vi "leybold QMH german.vi"() -> ()   [LabVIEW 2023]
uses:
  usr/local/natinst/LabVIEW-2023-64/examples/Design Patterns/Queued Message Handler/support/QMH Fundamentals - Message Cluster.ctl
  <vilib>/Instr/_visa.llb/VISA Configure Serial Port (Instr).vi
  global variables.vi
  <vilib>/Utility/error.llb/Error Cluster From Error Code.vi
  SubVI library/Send Graphite Metrics/Send Graphite Metrics.vi
  <vilib>/ErrorRing/Error Ring.xnode
panel:
  out "unsigned byte array":u8[](array[numeric])
  in  "Stop":bool
  in  "recipes":bool
  in  "Tab Control":T1(tab)
  out "REF Leistung (W)":i16
  in  "Vorwartsleistung (W)":bool=TRUE
  in  "CL":bool
  in  "CT":bool
  in  "RF Quelle":bool
  out "PFG600":string
  out "Antwort":string
  in  "+100":bool
  out "DC Spannung (V)":i16
  in  "Argon (SCCM)":bool
  in  "Sauerstioff (SCCM)":bool
  in  "Gas":bool
  in  "+10":bool
  in  "+1":bool
  in  "-1":bool
  in  "-10":bool
  in  "-100":bool
  in  "GAS Boost":bool
  in  "Timer":bool
  in  "Matchbox-Modus":bool
  in  "TimerOn":bool
  out "PR4000":string
  in  "P1":bool
  in  "P2":bool
  in  "P3":bool
  out "Endzeit":timestamp format="%<%H:%M:%S>T"
  out "Time":timestamp format="%<%H:%M:%S\n%x>T"
  in  "RS232":bool
  out "Waveform Chart":waveform(dbl)(graph)
  in  "1h":bool
  in  "8h":bool
  in  "24h":bool
  in  "All":bool
  out "Druck (mbar)":dbl format="%#_6e"
  # "GENERATOR"
  # "MFC"
  # "TIMER"
  # "VOREINSTELLUNGEN"
  # "DEBUG"
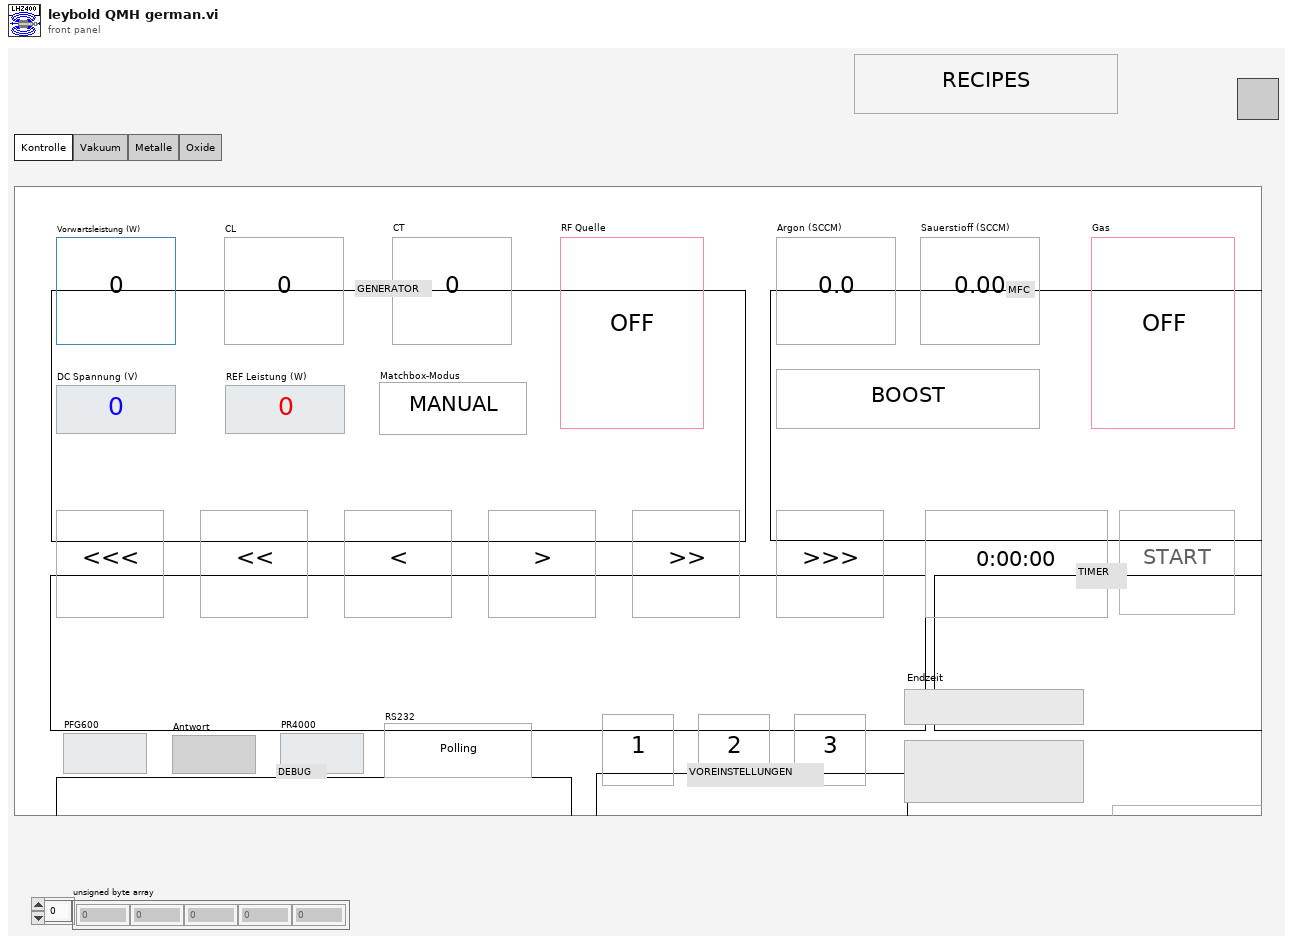
[diagram p1: front panel]
types:
  T1 = enum32{"Kontrolle", "Vakuum", "Metalle", "Oxide"}
  T2 = typedef "QMH Fundamentals - Message Cluster.ctl" = cluster{"Message":string, "Message Data":variant}
  T3 = cluster{"Message":string, enum16{"FWD", "CL", "CT", "Ar", "O2", "Timer"}}
  T4 = enum8{"Enabled", "Disabled", "Disabled and Grayed Out"}
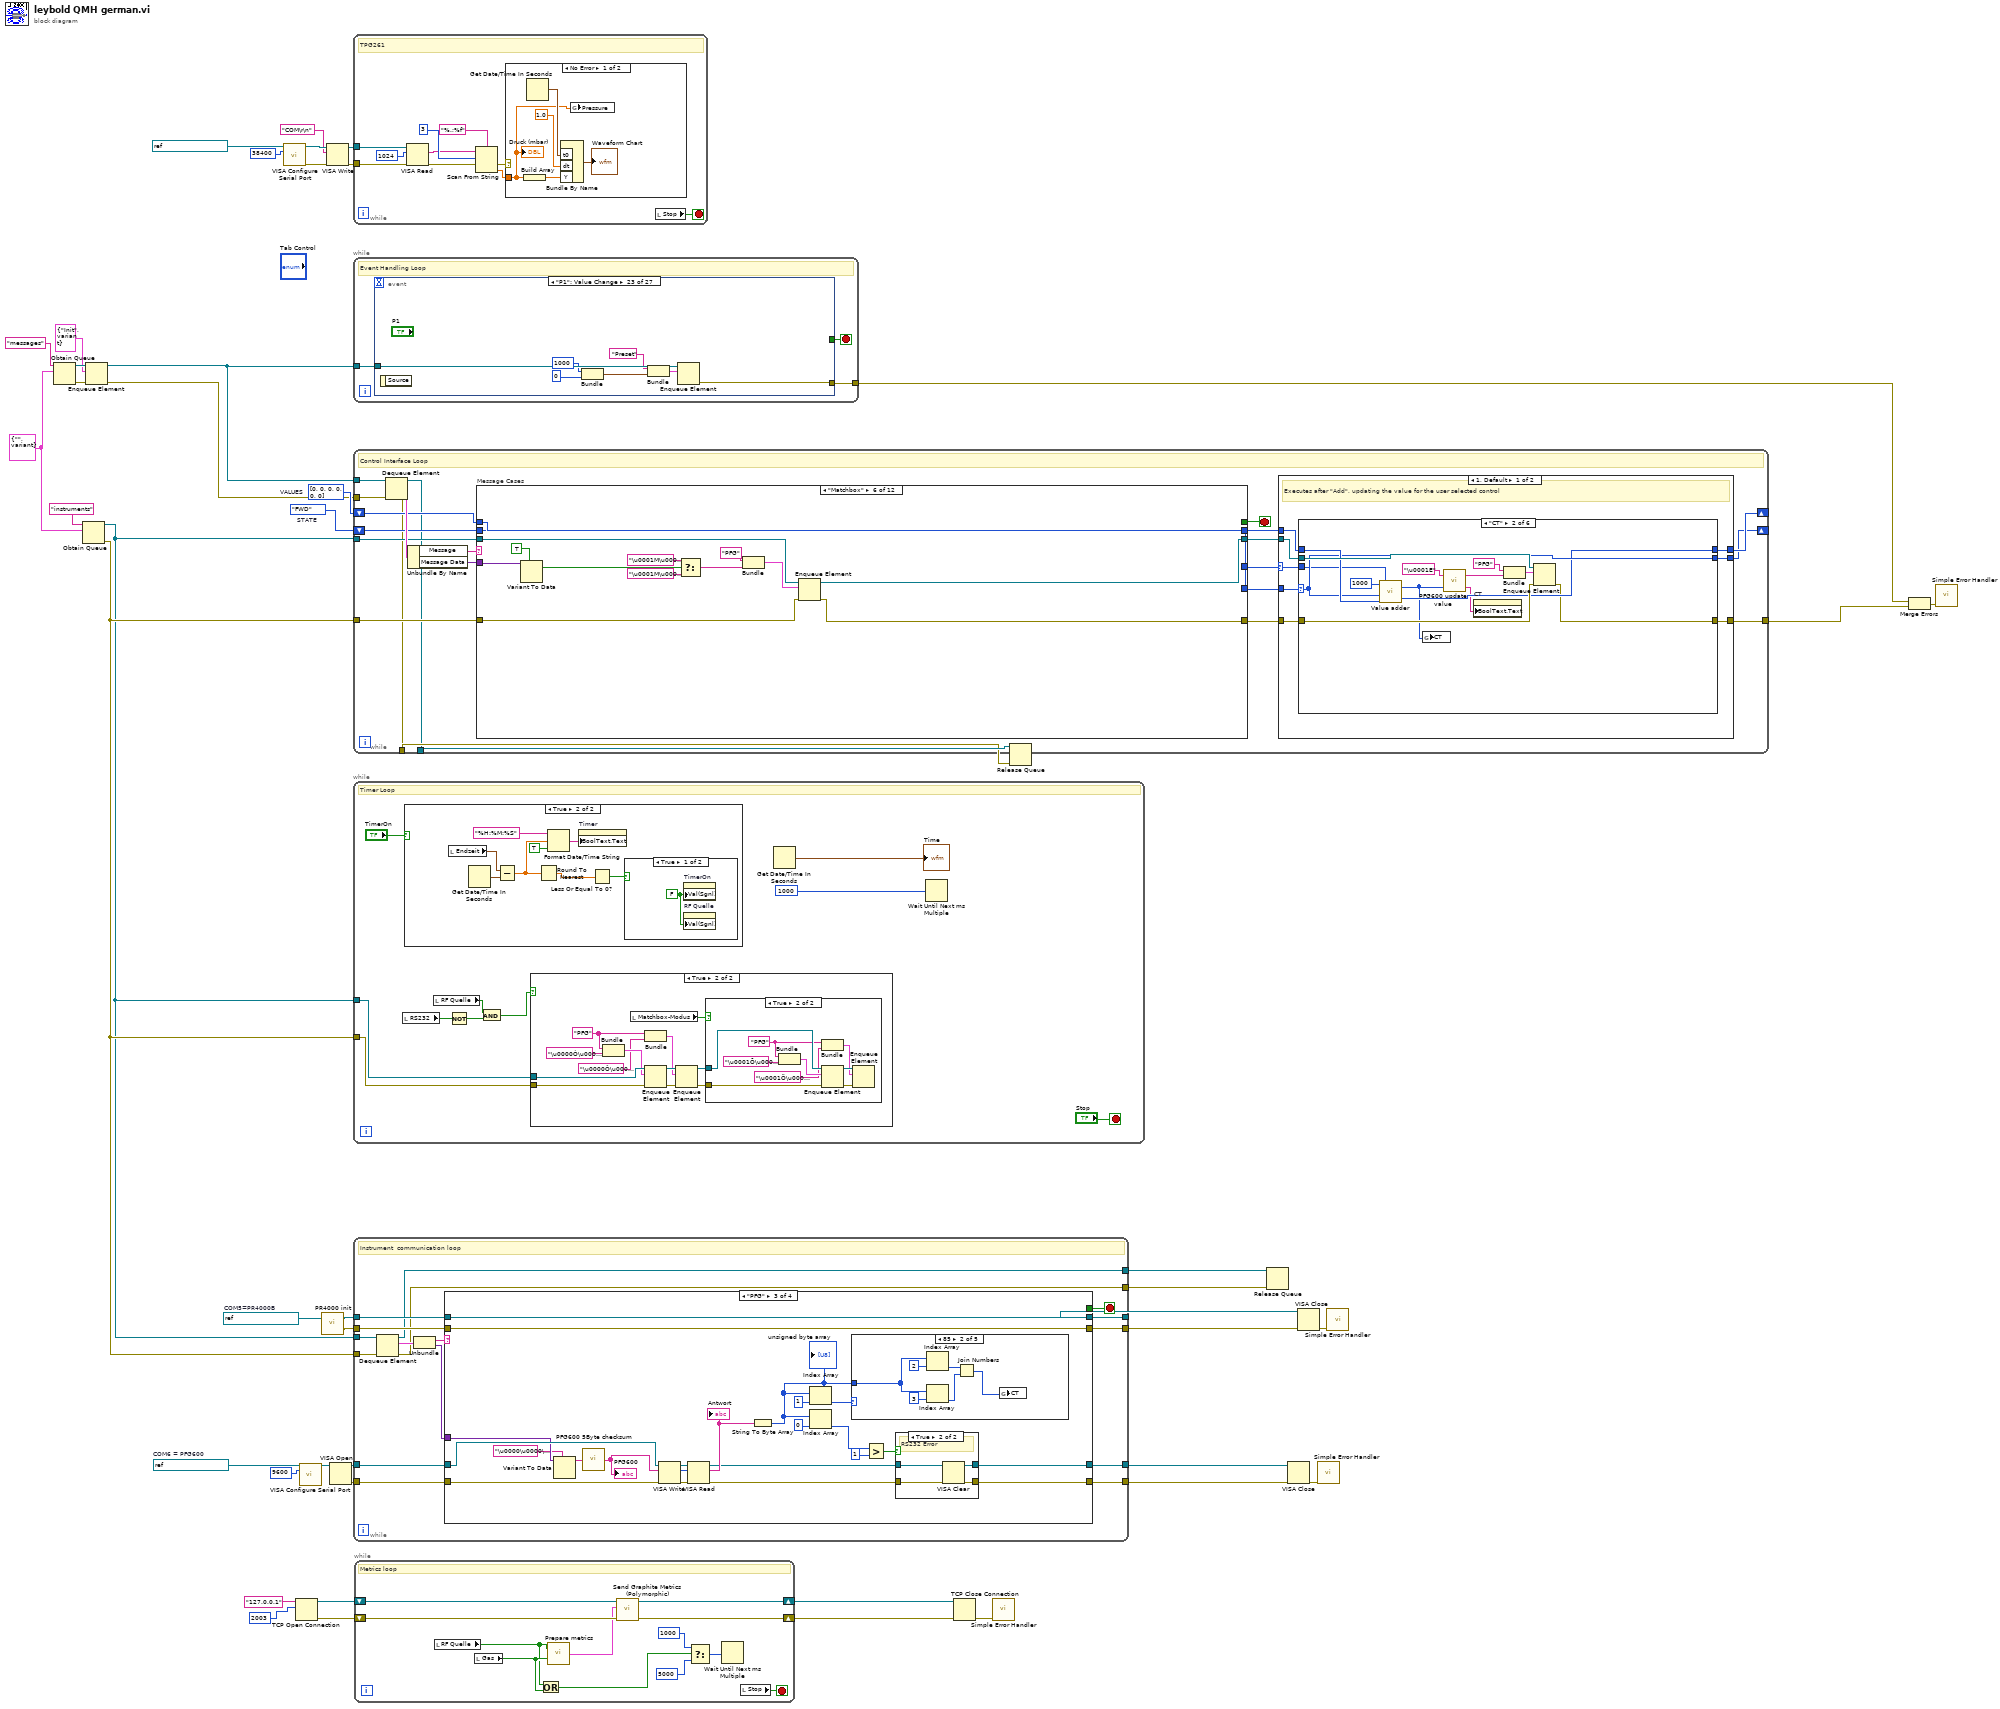
[diagram p0: block diagram]
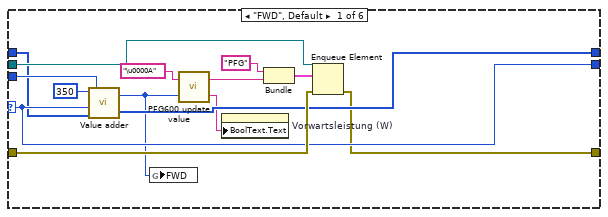
[diagram p6: hidden frame]
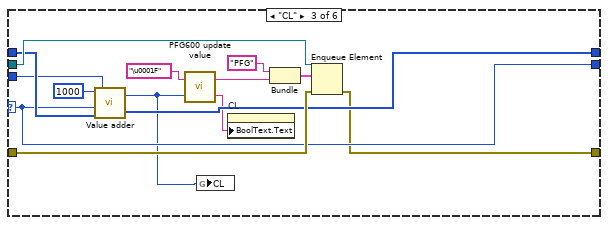
[diagram p7: hidden frame]
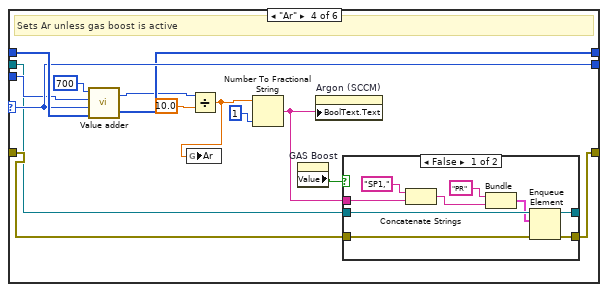
[diagram p8: hidden frame]
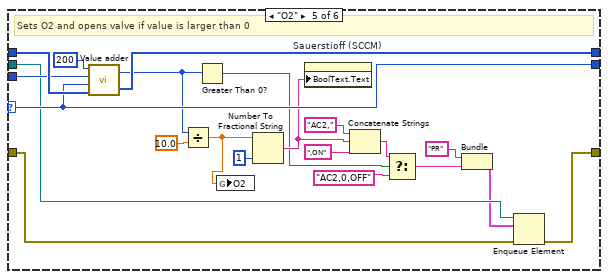
[diagram p10: hidden frame]
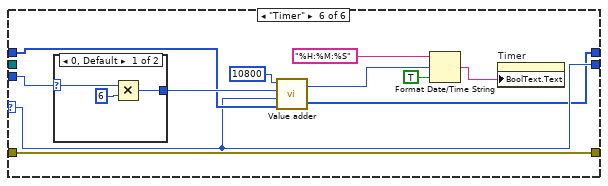
[diagram p11: hidden frame]
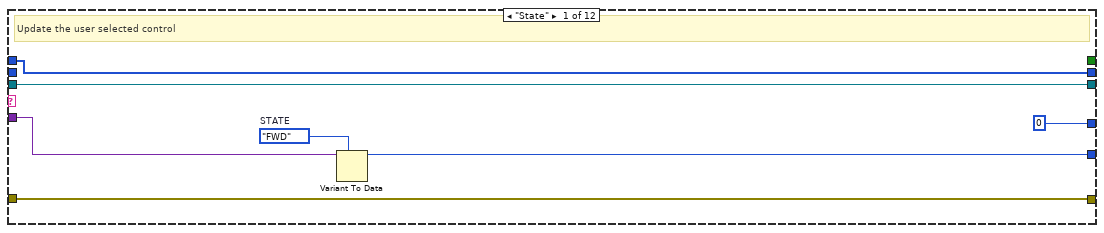
[diagram p14: hidden frame]
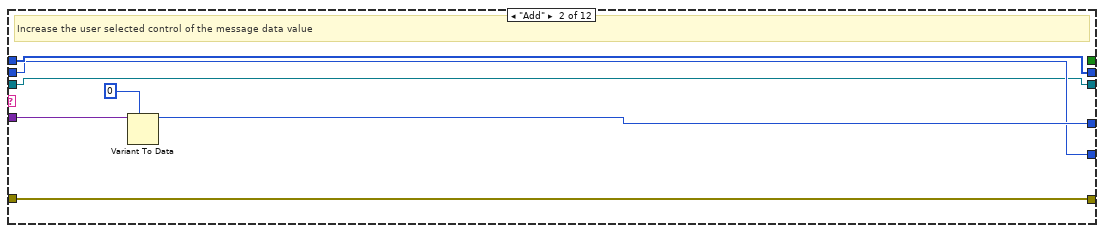
[diagram p15: hidden frame]
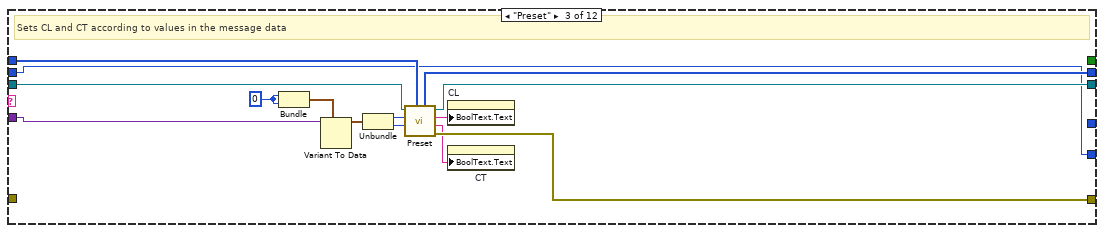
[diagram p16: hidden frame]
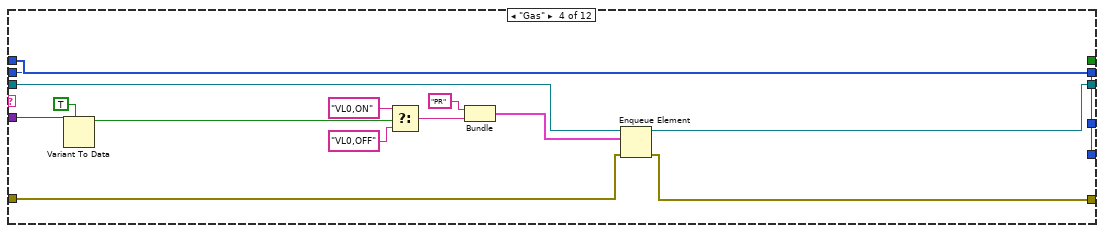
[diagram p17: hidden frame]
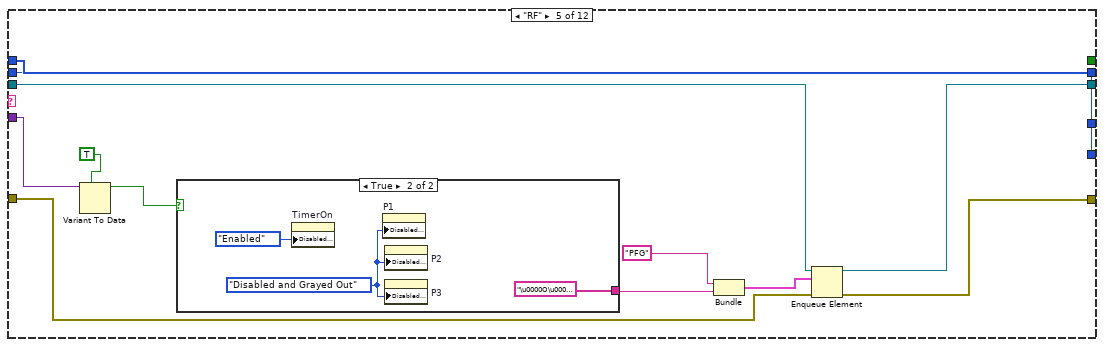
[diagram p18: hidden frame]
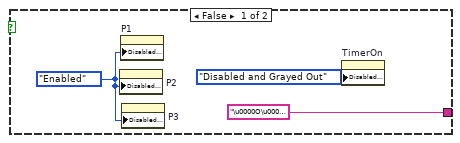
[diagram p19: hidden frame]
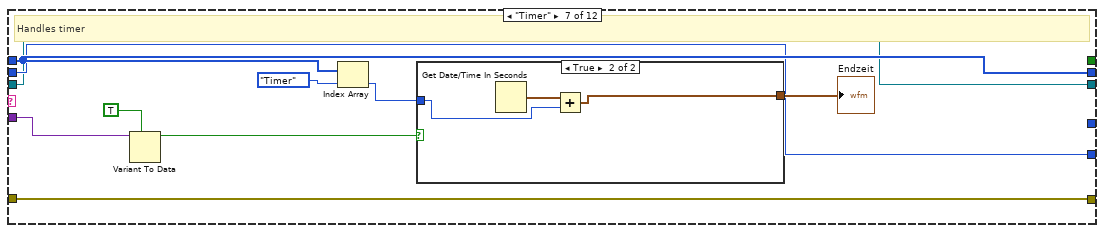
[diagram p20: hidden frame]
diagram:
  w27 = i16[] [0, 0, 0, 0, 0, 0]  # VALUES
  w28 = enum16{"FWD", "CL", "CT", "Ar", "O2", "Timer"}."FWD"  # STATE
  w19 = T2 {"Message"="", "Message Data"=variant} ("Message Cluster")
  w41 = refnum<visa-resource-name> "ASRL34::INSTR"  # COM5=PR4000B
  w15 = refnum<visa-resource-name> "ASRL36::INSTR"  # COM6 = PFG600
  n1 = Obtain Queue(name (unnamed)="messages", element data type=w19) -> (queue out=w32:refnum<queue>, error out=w33:errorcluster)  [unwired: 3 in, 1 out]
  n2 = Obtain Queue(name (unnamed)="instruments", element data type=w19) -> (queue out=w1:refnum<queue>, error out=w2:errorcluster)  [unwired: 3 in, 1 out]
  n3 = Enqueue Element(queue=w32, element=T2 {"Message"="Init", "Message Data"=variant}, error in (no error)=w33) -> (queue out=w26:refnum<queue>, error out=w10:errorcluster)  [unwired: 1 in, 1 out]
  n4 = call-poly "VISA Configure Serial Port"("VISA resource name"=refnum<visa-resource-name> "ASRL33::INSTR", "baud rate (9600)"=u32 38400) -> ("VISA resource name out"=w36:refnum<visa-resource-name>, "error out"=w37:errorcluster)  [unwired: 12 in]
  n5 = TCP Open Connection(address="127.0.0.1", remote port or service name=u16 2003) -> (connection ID=w7:refnum<k5>, error out=w6:errorcluster)  [unwired: 3 in]
  n6 = call-poly "VISA Configure Serial Port"("VISA resource name"=w15, "baud rate (9600)"=u32 9600) -> ("VISA resource name out"=w16:refnum<visa-resource-name>)  [unwired: 12 in, 1 out]
  n7 = call "PR4000 init.vi"("VISA Refnum in"=w41) -> ("error out"=w24:errorcluster, "VISA Refnum out"=w25:refnum<visa-resource-name>)  [unwired: 1 in]
  n8 = VISA Write(VISA resource name=w36, write buffer="COM\r\n", error in (no error)=w37) -> (VISA resource name out=w38:refnum<visa-resource-name>, error out=w34:errorcluster)  [unwired: 1 out]
  n9 = VISA Open(VISA resource name=w16) -> (VISA resource name=w46:refnum<visa-resource-name>, error out=w47:errorcluster)  [unwired: 4 in]
  n10 = while {
    tunnel: w38 -> [w57]
    tunnel: w34 -> [w56]
    stop <- w48 stop-if-true
    # "TPG261"
    n11 = VISA Read(VISA resource name=w57, byte count=u32 1024, error in (no error)=w56) -> (read buffer=w52:string, error out=w50:errorcluster)  [unwired: 2 out]
    n12 = Scan From String(format string="%.;%f" ("Format-String"), input string=w52, initial scan location=u32 3 ("offset (0)"), error in=w50) -> (error out=w49:errorcluster, output 1=w51:dbl)  [unwired: 1 in, 2 out]
    n13 = case shown="No Error" w49 {
      tunnel: w51 -> [w58 _]
      frame No Error {
        n14 = Build Array(w58) -> (w62:dbl[])
        n15 = Get Date/Time In Seconds() -> (seconds since 1Jan1904=w59:timestamp)
        n16 = Bundle By Name("t0"=w59, "dt"=1.0, "Y"=w62) -> (→"Waveform Chart":waveform(dbl))  [unwired: 1 in]
        n17 = global write "global variables.vi" "Pressure"(w58) -> ()
        "Druck (mbar)" <- w58
      }
      frame Error {
      }
    }
    n18 = local read "Stop"() -> (w48:bool)
  }
  n19 = while {
    tunnel: w26 -> [w65]
    tunnel: [w63] -> w30
    stop <- w64 stop-if-true
    # "Event Handling Loop"
    n20 = event shown="[22] \"P1\": Value Change" {
      selector: _ -> [_ _ _ _ _ _ _ _ _ _ _ _ _ _ _ _ _ _ _ _ _ _ _ _ _ _ _]
      dyn-events: _ -> [_ _ _ _ _ _ _ _ _ _ _ _ _ _ _ _ _ _ _ _ _ _ _ _ _ _ _]
      timeout: _ -> [_ _ _ _ _ _ _ _ _ _ _ _ _ _ _ _ _ _ _ _ _ _ _ _ _ _ _]
      tunnel: [TRUE _ _ _ _ _ _ _ _ _ _ _ _ _ _ _ _ _ _ _ _ _ _ _ _ _ _] -> w64
      tunnel: w65 -> [w69 w71 w76 w81 w86 w91 w98 w103 w108 w113 w118 w122 w125 w128 w131 w134 w137 w142 w147 _ w156 w160 w168 w175 w182 w187 _]
      tunnel: [w68 w70 w75 w80 w85 w90 w95 w100 w105 w110 w115 w121 w124 w127 w130 w133 w136 w141 w146 _ w152 w157 w162 w169 w176 w186 _] -> w63
      event "Stop": Value Change {
        # "Stop the VI."
        # "Enqueue an \"Exit\" message. Note that the Enqueue Element At Opposite End function is used to place this priority \"Exit\" message at the front of the queue ahead of all other messages."
        n21 = event-data() -> ()  [unwired: 1 in, 1 out]
        n22 = Enqueue Element At Opposite End(queue=w69, element=T2 {"Message"="Exit", "Message Data"=variant}) -> (error out=w68:errorcluster)  [unwired: 2 in, 2 out]
      }
      event "1h": Value Change {
        n23 = event-data() -> ()  [unwired: 1 in, 1 out]
        n24 = Bundle("Scale", 3600) -> (w73:cluster{string, i32})  [unwired: 1 in]
        n25 = Enqueue Element(queue=w71, element=w73) -> (error out=w70:errorcluster)  [unwired: 2 in, 2 out]
      }
      event "8h": Value Change {
        n26 = event-data() -> ()  [unwired: 1 in, 1 out]
        n27 = Bundle("Scale", 28800) -> (w78:cluster{string, i32})  [unwired: 1 in]
        n28 = Enqueue Element(queue=w76, element=w78) -> (error out=w75:errorcluster)  [unwired: 2 in, 2 out]
      }
      event "24h": Value Change {
        n29 = event-data() -> ()  [unwired: 1 in, 1 out]
        n30 = Bundle("Scale", 86400) -> (w83:cluster{string, i32})  [unwired: 1 in]
        n31 = Enqueue Element(queue=w81, element=w83) -> (error out=w80:errorcluster)  [unwired: 2 in, 2 out]
      }
      event "All": Value Change {
        n32 = event-data() -> ()  [unwired: 1 in, 1 out]
        n33 = Bundle("Scale", 0) -> (w88:cluster{string, i32})  [unwired: 1 in]
        n34 = Enqueue Element(queue=w86, element=w88) -> (error out=w85:errorcluster)  [unwired: 2 in, 2 out]
      }
      event "CL": Value Change {
        w94 = FALSE ("FWD Power (W)")
        n35 = event-data() -> ()  [unwired: 1 in, 1 out]
        n36 = Enqueue Element(queue=w91, element=T3 {"Message"="State", enum."CL"}) -> (error out=w90:errorcluster)  [unwired: 2 in, 2 out]
        n37 = property on="CT" class="Bool (strict)"("Value"=w94) -> ()  [unwired: 2 in, 2 out]
        n38 = property on="Timer" class="Bool (strict)"("Value"=w94) -> ()  [unwired: 2 in, 2 out]
        n39 = property on="CL" class="Bool (strict)"("Value"=TRUE ("CL")) -> ()  [unwired: 2 in, 2 out]
        n40 = property on="Argon (SCCM)" class="Bool (strict)"("Value"=w94) -> ()  [unwired: 2 in, 2 out]
        n41 = property on="Sauerstioff (SCCM)" class="Bool (strict)"("Value"=w94) -> ()  [unwired: 2 in, 2 out]
        n42 = property on="Vorwartsleistung (W)" class="Bool (strict)"("Value"=w94) -> ()  [unwired: 2 in, 2 out]
      }
      event "CT": Value Change {
        w97 = FALSE ("FWD Power (W)")
        n43 = event-data() -> ()  [unwired: 1 in, 1 out]
        n44 = Enqueue Element(queue=w98, element=T3 {"Message"="State", enum."CT"}) -> (error out=w95:errorcluster)  [unwired: 2 in, 2 out]
        n45 = property on="CT" class="Bool (strict)"("Value"=TRUE ("CL")) -> ()  [unwired: 2 in, 2 out]
        n46 = property on="CL" class="Bool (strict)"("Value"=w97) -> ()  [unwired: 2 in, 2 out]
        n47 = property on="Timer" class="Bool (strict)"("Value"=w97) -> ()  [unwired: 2 in, 2 out]
        n48 = property on="Argon (SCCM)" class="Bool (strict)"("Value"=w97) -> ()  [unwired: 2 in, 2 out]
        n49 = property on="Sauerstioff (SCCM)" class="Bool (strict)"("Value"=w97) -> ()  [unwired: 2 in, 2 out]
        n50 = property on="Vorwartsleistung (W)" class="Bool (strict)"("Value"=w97) -> ()  [unwired: 2 in, 2 out]
      }
      event "Argon (SCCM)": Value Change {
        w102 = FALSE ("FWD Power (W)")
        n51 = event-data() -> ()  [unwired: 1 in, 1 out]
        n52 = Enqueue Element(queue=w103, element=T3 {"Message"="State", enum."Ar"}) -> (error out=w100:errorcluster)  [unwired: 2 in, 2 out]
        n53 = property on="CL" class="Bool (strict)"("Value"=w102) -> ()  [unwired: 2 in, 2 out]
        n54 = property on="Argon (SCCM)" class="Bool (strict)"("Value"=TRUE ("CL")) -> ()  [unwired: 2 in, 2 out]
        n55 = property on="Timer" class="Bool (strict)"("Value"=w102) -> ()  [unwired: 2 in, 2 out]
        n56 = property on="CT" class="Bool (strict)"("Value"=w102) -> ()  [unwired: 2 in, 2 out]
        n57 = property on="Sauerstioff (SCCM)" class="Bool (strict)"("Value"=w102) -> ()  [unwired: 2 in, 2 out]
        n58 = property on="Vorwartsleistung (W)" class="Bool (strict)"("Value"=w102) -> ()  [unwired: 2 in, 2 out]
      }
      event "Sauerstioff (SCCM)": Value Change {
        w107 = FALSE ("FWD Power (W)")
        n59 = event-data() -> ()  [unwired: 1 in, 1 out]
        n60 = Enqueue Element(queue=w108, element=T3 {"Message"="State", enum."O2"}) -> (error out=w105:errorcluster)  [unwired: 2 in, 2 out]
        n61 = property on="CL" class="Bool (strict)"("Value"=w107) -> ()  [unwired: 2 in, 2 out]
        n62 = property on="Sauerstioff (SCCM)" class="Bool (strict)"("Value"=TRUE ("CL")) -> ()  [unwired: 2 in, 2 out]
        n63 = property on="Timer" class="Bool (strict)"("Value"=w107) -> ()  [unwired: 2 in, 2 out]
        n64 = property on="CT" class="Bool (strict)"("Value"=w107) -> ()  [unwired: 2 in, 2 out]
        n65 = property on="Argon (SCCM)" class="Bool (strict)"("Value"=w107) -> ()  [unwired: 2 in, 2 out]
        n66 = property on="Vorwartsleistung (W)" class="Bool (strict)"("Value"=w107) -> ()  [unwired: 2 in, 2 out]
      }
      event "Vorwartsleistung (W)": Value Change {
        w112 = FALSE ("FWD Power (W)")
        n67 = event-data() -> ()  [unwired: 1 in, 1 out]
        n68 = Enqueue Element(queue=w113, element=T3 {"Message"="State", enum."FWD"}) -> (error out=w110:errorcluster)  [unwired: 2 in, 2 out]
        n69 = property on="Vorwartsleistung (W)" class="Bool (strict)"("Value"=TRUE ("CL")) -> ()  [unwired: 2 in, 2 out]
        n70 = property on="Sauerstioff (SCCM)" class="Bool (strict)"("Value"=w112) -> ()  [unwired: 2 in, 2 out]
        n71 = property on="Timer" class="Bool (strict)"("Value"=w112) -> ()  [unwired: 2 in, 2 out]
        n72 = property on="CL" class="Bool (strict)"("Value"=w112) -> ()  [unwired: 2 in, 2 out]
        n73 = property on="Argon (SCCM)" class="Bool (strict)"("Value"=w112) -> ()  [unwired: 2 in, 2 out]
        n74 = property on="CT" class="Bool (strict)"("Value"=w112) -> ()  [unwired: 2 in, 2 out]
      }
      event "Timer": Value Change {
        w116 = FALSE ("FWD Power (W)")
        n75 = event-data() -> ()  [unwired: 1 in, 1 out]
        n76 = Enqueue Element(queue=w118, element=T3 {"Message"="State", enum."Timer"}) -> (error out=w115:errorcluster)  [unwired: 2 in, 2 out]
        n77 = property on="CT" class="Bool (strict)"("Value"=w116) -> ()  [unwired: 2 in, 2 out]
        n78 = property on="Timer" class="Bool (strict)"("Value"=TRUE ("CL")) -> ()  [unwired: 2 in, 2 out]
        n79 = property on="CL" class="Bool (strict)"("Value"=w116) -> ()  [unwired: 2 in, 2 out]
        n80 = property on="Argon (SCCM)" class="Bool (strict)"("Value"=w116) -> ()  [unwired: 2 in, 2 out]
        n81 = property on="Sauerstioff (SCCM)" class="Bool (strict)"("Value"=w116) -> ()  [unwired: 2 in, 2 out]
        n82 = property on="Vorwartsleistung (W)" class="Bool (strict)"("Value"=w116) -> ()  [unwired: 2 in, 2 out]
      }
      event "-100": Value Change {
        n83 = event-data() -> ()  [unwired: 1 in, 1 out]
        n84 = Enqueue Element(queue=w122, element=cluster{"Message":string, i32} {"Message"="Add", -100}) -> (error out=w121:errorcluster)  [unwired: 2 in, 2 out]
      }
      event "-10": Value Change {
        n85 = event-data() -> ()  [unwired: 1 in, 1 out]
        n86 = Enqueue Element(queue=w125, element=cluster{"Message":string, i32} {"Message"="Add", -10}) -> (error out=w124:errorcluster)  [unwired: 2 in, 2 out]
      }
      event "-1": Value Change {
        n87 = event-data() -> ()  [unwired: 1 in, 1 out]
        n88 = Enqueue Element(queue=w128, element=cluster{"Message":string, i32} {"Message"="Add", -1}) -> (error out=w127:errorcluster)  [unwired: 2 in, 2 out]
      }
      event "+1": Value Change {
        n89 = event-data() -> ()  [unwired: 1 in, 1 out]
        n90 = Enqueue Element(queue=w131, element=cluster{"Message":string, i32} {"Message"="Add", 1}) -> (error out=w130:errorcluster)  [unwired: 2 in, 2 out]
      }
      event "+10": Value Change {
        n91 = event-data() -> ()  [unwired: 1 in, 1 out]
        n92 = Enqueue Element(queue=w134, element=cluster{"Message":string, i32} {"Message"="Add", 10}) -> (error out=w133:errorcluster)  [unwired: 2 in, 2 out]
      }
      event "+100": Value Change {
        n93 = event-data() -> ()  [unwired: 1 in, 1 out]
        n94 = Enqueue Element(queue=w137, element=cluster{"Message":string, i32} {"Message"="Add", 100}) -> (error out=w136:errorcluster)  [unwired: 2 in, 2 out]
      }
      event "GAS Boost": Value Change {
        n95 = event-data() -> ()  [unwired: 1 in, 1 out]
        n96 = Bundle("Message"="Boost", "GAS Boost"="GAS Boost") -> (w138:cluster{"Message":string, "GAS Boost":bool})  [unwired: 1 in]
        n97 = Enqueue Element(queue=w142, element=w138) -> (error out=w141:errorcluster)  [unwired: 2 in, 2 out]
      }
      event "Gas": Value Change {
        n98 = event-data() -> ()  [unwired: 1 in, 1 out]
        n99 = Bundle("Gas", "Gas"="Gas") -> (w145:cluster{string, "Gas":bool})  [unwired: 1 in]
        n100 = Enqueue Element(queue=w147, element=w145) -> (error out=w146:errorcluster)  [unwired: 2 in, 2 out]
      }
      event "RS232": Value Change {
        n101 = event-data() -> ()  [unwired: 1 in, 1 out]
        n102 = case shown="True" "RS232" {
          tunnel: [T4."Enabled" ("Disabled") T4."Disabled and Grayed Out" ("Disabled")] -> w148
          frame False {
          }
          frame True {
          }
        }
        n103 = property on="DC Spannung (V)" class="DigNum (strict)"("DisabledEnum"=w148) -> ()  [unwired: 2 in, 2 out]
        n104 = property on="REF Leistung (W)" class="DigNum (strict)"("DisabledEnum"=w148) -> ()  [unwired: 2 in, 2 out]
      }
      event "TimerOn": Value Change {
        n105 = event-data() -> ("NewVal"=w155:bool)  [unwired: 1 in]
        n106 = Bundle("Timer", "NewVal"=w155) -> (w153:cluster{string, "NewVal":bool})  [unwired: 1 in]
        n107 = Enqueue Element(queue=w156, element=w153) -> (error out=w152:errorcluster)  [unwired: 2 in, 2 out]
      }
      event "RF Quelle": Value Change {
        n108 = event-data() -> ()  [unwired: 1 in, 1 out]
        n109 = Bundle("RF", "RF Quelle"="RF Quelle") -> (w159:cluster{string, "RF Quelle":bool})  [unwired: 1 in]
        n110 = Enqueue Element(queue=w160, element=w159) -> (error out=w157:errorcluster)  [unwired: 2 in, 2 out]
      }
      event "P1": Value Change {
        n111 = event-data() -> ()  [unwired: 1 in, 1 out]
        n112 = Bundle(1000, 0) -> (w165:cluster{i32, i32})  [unwired: 1 in]
        n113 = Bundle("Preset", w165) -> (w166:cluster{string, cluster{i32, i32}})  [unwired: 1 in]
        n114 = Enqueue Element(queue=w168, element=w166) -> (error out=w162:errorcluster)  [unwired: 2 in, 2 out]
      }
      event "P2": Value Change {
        n115 = event-data() -> ()  [unwired: 1 in, 1 out]
        n116 = Bundle(250, 750) -> (w172:cluster{i32, i32})  [unwired: 1 in]
        n117 = Bundle("Preset", w172) -> (w173:cluster{string, cluster{i32, i32}})  [unwired: 1 in]
        n118 = Enqueue Element(queue=w175, element=w173) -> (error out=w169:errorcluster)  [unwired: 2 in, 2 out]
      }
      event "P3": Value Change {
        n119 = event-data() -> ()  [unwired: 1 in, 1 out]
        n120 = Bundle(680, 580) -> (w179:cluster{i32, i32})  [unwired: 1 in]
        n121 = Bundle("Preset", w179) -> (w180:cluster{string, cluster{i32, i32}})  [unwired: 1 in]
        n122 = Enqueue Element(queue=w182, element=w180) -> (error out=w176:errorcluster)  [unwired: 2 in, 2 out]
      }
      event "Matchbox-Modus": Value Change {
        n123 = event-data() -> ()  [unwired: 1 in, 1 out]
        n124 = Bundle("Matchbox", "Matchbox-Modus"="Matchbox-Modus") -> (w183:cluster{string, "Matchbox-Modus":bool})  [unwired: 1 in]
        n125 = Enqueue Element(queue=w187, element=w183) -> (error out=w186:errorcluster)  [unwired: 2 in, 2 out]
      }
      event "recipes": Value Change {
        n126 = event-data() -> ()  [unwired: 1 in, 1 out]
        n127 = call <vilib>:"System Exec.vi"("wait until completion? (T)"=FALSE, "command line"="firefox https://docs.google.com/spreadsheets/d/1f53240c20IwFszMSA94HhWp93EeL4Y7tCwhda4_pTaQ/edit#gid=1759381600 ") -> ()  [unwired: 6 in, 4 out]
      }
    }
  }
  n128 = while {
    tunnel: w26 -> [w206]
    tunnel: w10 -> [w205]
    shift-right: [w202] -> _
    shift-left: w27 -> [w201]
    shift-right: [w196] -> _
    shift-left: w28 -> [w204]
    tunnel: w1 -> [w195]
    tunnel: [w193] -> w18
    tunnel: w2 -> [w192]
    tunnel: [w191] -> w14
    tunnel: [w190] -> w13
    stop <- w194 stop-if-true
    # "Control Interface Loop"
    n129 = Dequeue Element(queue=w206, error in (no error)=w205) -> (queue out=w191:refnum<queue>, element=w209:T2, error out=w190:errorcluster)  [unwired: 1 in, 1 out]
    n130 = Unbundle By Name(w209) -> ("Message"=w208:string, "Message Data"=w207:variant)
    n131 = case "Message Cases" shown="\"Matchbox\"" w208 {
      selector: w208 -> [_ _ _ _ _ _ _ _ _ w450 _ w472]
      tunnel: w207 -> [w330 w337 w351 w361 w369 w389 w403 w426 _ w449 w464 _]
      tunnel: [w327 w334 w342 w365 w377 w397 w401 w424 w446 w456 w470 w476] -> w198
      tunnel: w204 -> [_ w333 w339 w364 w376 w396 w400 w417 w445 w455 w467 w475]
      tunnel: [0 w335 _ _ _ _ _ 0 _ _ _ 0] -> w203
      tunnel: w201 -> [w327 w334 w343 w365 w377 w397 w401 w424 w446 w456 w470 w476]
      tunnel: [w325 w332 w345 w357 w370 w393 w399 w420 w444 w453 w469 w474] -> w200
      tunnel: [w324 w331 w344 w362 w371 w392 w398 w419 w438 w447 w468 w471] -> w199
      tunnel: [w326 w333 w339 w364 w376 w396 w400 w417 w445 w455 w467 w475] -> w197
      tunnel: w195 -> [w325 w332 w338 w363 w372 w394 w399 w416 w444 w452 w469 w474]
      tunnel: [_ _ _ _ _ _ _ _ _ TRUE _ _] -> w194
      tunnel: w192 -> [w324 w331 _ w356 w366 w388 w398 _ w438 w448 w468 w471]
      frame "State" {
        w328 = enum16{"FWD", "CL", "CT", "Ar", "O2", "Timer"}."FWD"  # STATE
        # "Update the user selected control"
        n132 = Variant To Data(type=w328, Variant=w330) -> (data=w326:enum16{"FWD", "CL", "CT", "Ar", "O2", "Timer"})  [unwired: 1 in, 1 out]
      }
      frame "Add" {
        # "Increase the user selected control of the message data value"
        n133 = Variant To Data(type=0, Variant=w337) -> (data=w335:i32)  [unwired: 1 in, 1 out]
      }
      frame "Preset" {
        w350 = 0
        # "Sets CL and CT according to values in the message data"
        n134 = Bundle(w350, w350) -> (w349:cluster{i32, i32})  [unwired: 1 in]
        n135 = Variant To Data(type=w349, Variant=w351) -> (data=w348:cluster{i32, i32})  [unwired: 1 in, 1 out]
        n136 = Unbundle(w348) -> (w347:i32, w346:i32)
        n137 = call "Preset.vi"("Array"=w343, "CT"=w346, "CL"=w347, "queue in"=w338) -> ("error out"=w344:errorcluster, "Text CT"=w340:string, "Text CL"=w341:string, "queue out"=w345:refnum<queue>, "output array"=w342:i16[])  [unwired: 3 in]
        n138 = property on="CL" class="Bool (strict)"("BoolText.Text"=w341) -> ()  [unwired: 2 in, 2 out]
        n139 = property on="CT" class="Bool (strict)"("BoolText.Text"=w340) -> ()  [unwired: 2 in, 2 out]
      }
      frame "Gas" {
        n140 = Variant To Data(type=TRUE, Variant=w361) -> (data=w355:bool)  [unwired: 1 in, 1 out]
        n141 = Select(t="VL0,ON" ("string"), s=w355, f="VL0,OFF" ("string")) -> (s? t:f=w352:string)
        n142 = Bundle("PR", "string"=w352) -> (w358:cluster{string, "string":string})  [unwired: 1 in]
        n143 = Enqueue Element(queue=w363, element=w358, error in (no error)=w356) -> (queue out=w357:refnum<queue>, error out=w362:errorcluster)  [unwired: 1 in, 1 out]
      }
      frame "RF" {
        n144 = Variant To Data(type=TRUE, Variant=w369) -> (data=w367:bool)  [unwired: 1 in, 1 out]
        n145 = case shown="True" w367 {
          tunnel: ["\u0000O\u0000\u0000" "\u0000O\u0000\u0001"] -> w375
          frame False {
            w378 = T4."Enabled" ("Disabled")
            n146 = property on="P2" class="Bool"("DisabledEnum"=w378) -> ()  [unwired: 2 in, 2 out]
            n147 = property on="P1" class="Bool"("DisabledEnum"=w378) -> ()  [unwired: 2 in, 2 out]
            n148 = property on="P3" class="Bool"("DisabledEnum"=w378) -> ()  [unwired: 2 in, 2 out]
            n149 = property on="TimerOn" class="Bool (strict)"("DisabledEnum"=T4."Disabled and Grayed Out" ("Disabled")) -> ()  [unwired: 2 in, 2 out]
          }
          frame True {
            w381 = T4."Disabled and Grayed Out" ("Disabled")
            n150 = property on="TimerOn" class="Bool (strict)"("DisabledEnum"=T4."Enabled" ("Disabled")) -> ()  [unwired: 2 in, 2 out]
            n151 = property on="P1" class="Bool"("DisabledEnum"=w381) -> ()  [unwired: 2 in, 2 out]
            n152 = property on="P2" class="Bool"("DisabledEnum"=w381) -> ()  [unwired: 2 in, 2 out]
            n153 = property on="P3" class="Bool"("DisabledEnum"=w381) -> ()  [unwired: 2 in, 2 out]
          }
        }
        n154 = Bundle("PFG", w375) -> (w373:cluster{string, string})  [unwired: 1 in]
        n155 = Enqueue Element(queue=w372, element=w373, error in (no error)=w366) -> (queue out=w370:refnum<queue>, error out=w371:errorcluster)  [unwired: 1 in, 1 out]
      }
      frame "Matchbox" {
        n156 = Variant To Data(type=TRUE, Variant=w389) -> (data=w387:bool)  [unwired: 1 in, 1 out]
        n157 = Select(t="\u0001M\u0000\u0002", s=w387, f="\u0001M\u0000\u0001") -> (s? t:f=w384:string)
        n158 = Bundle("PFG", w384) -> (w391:cluster{string, string})  [unwired: 1 in]
        n159 = Enqueue Element(queue=w394, element=w391, error in (no error)=w388) -> (queue out=w393:refnum<queue>, error out=w392:errorcluster)  [unwired: 1 in, 1 out]
      }
      frame "Timer" {
        # "Handles timer"
        n160 = Variant To Data(type=TRUE, Variant=w403) -> (data=w402:bool)  [unwired: 1 in, 1 out]
        n161 = Index Array(array=w401, index=enum16{"FWD", "CL", "CT", "Ar", "O2", "Timer"}."Timer") -> (element=w406:i16)
        n162 = case shown="True" w402 {
          tunnel: w406 -> [w408 w413]
          tunnel: [timestamp(0 s since 1904-01-01) w414] -> w407
          frame False {
            n163 = Format Date/Time String(time format string (%c)="%H:%M:%S", seconds (now)=w408, UTC format=TRUE) -> (date/time string=w409:string)
            n164 = property on="Timer" class="Bool (strict)"("BoolText.Text"=w409) -> ()  [unwired: 2 in, 2 out]
          }
          frame True {
            n165 = Get Date/Time In Seconds() -> (seconds since 1Jan1904=w415:timestamp)
            n166 = Add(x=w415, y=w413) -> (x+y=w414:timestamp)
          }
        }
        "Endzeit" <- w407
      }
      frame "Boost" {
        # "Sets Ar to 60 SCCM or revert to previous value"
        n167 = Variant To Data(type=TRUE, Variant=w426) -> (data=w418:bool)  [unwired: 1 in, 1 out]
        n168 = case shown="False" w418 {
          tunnel: [w433 "SP1,60.0"] -> w422
          tunnel: w424 -> [w436 _]
          frame False {
            n169 = Index Array(array=w436, index=enum16{"FWD", "CL", "CT", "Ar", "O2", "Timer"}."Ar") -> (element=w430:i16)
            n170 = Divide(x=w430, y=10.0) -> (x/y=w429:dbl)
            n171 = Number To Fractional String(number=w429, precision (6)=i16 1) -> (F-format string=w431:string)  [unwired: 2 in]
            n172 = Concatenate Strings("SP1," ("string"), w431) -> (w433:string)
          }
          frame True {
          }
        }
        n173 = Bundle("PR", w422) -> (w421:cluster{string, string})  [unwired: 1 in]
        n174 = Enqueue Element(queue=w416, element=w421) -> (queue out=w420:refnum<queue>, error out=w419:errorcluster)  [unwired: 2 in, 1 out]
      }
      frame "Init" {
        w439 = "0" ("Boolean Text.Text")
        # "Interface initzialization"
        n175 = property on="Tab Control" class="TabCtl (strict)"("TabHeight"=u32 50 ("Fixed Tab Dimension:Height")) -> ()  [unwired: 2 in, 2 out]
        n176 = property on="CL" class="Bool (strict)"("BoolText.Text"=w439) -> ()  [unwired: 2 in, 2 out]
        n177 = property on="Vorwartsleistung (W)" class="Bool (strict)"("BoolText.Text"=w439) -> ()  [unwired: 2 in, 2 out]
        n178 = property on="CT" class="Bool (strict)"("BoolText.Text"=w439) -> ()  [unwired: 2 in, 2 out]
        n179 = property on="Argon (SCCM)" class="Bool (strict)"("BoolText.Text"="0.0") -> ()  [unwired: 2 in, 2 out]
        n180 = invoke class="VI" method="Default Vals.Reinit All"() -> ()  [unwired: 3 in, 3 out]
        n181 = property on="Sauerstioff (SCCM)" class="Bool (strict)"("BoolText.Text"="0.00") -> ()  [unwired: 2 in, 2 out]
        n182 = property on="Timer" class="Bool (strict)"("BoolText.Text"="0:00:00" ("Boolean Text.Text")) -> ()  [unwired: 2 in, 2 out]
      }
      frame "Exit" {
        # "Stop the VI."
        # "Releases Queue and exit"
        n183 = Bundle(w450, "Message Data"=w449) -> (w451:cluster{string, "Message Data":variant})  [unwired: 1 in]
        n184 = Enqueue Element(queue=w452, element=w451, error in (no error)=w448) -> (queue out=w453:refnum<queue>, error out=w447:errorcluster)  [unwired: 1 in, 1 out]
      }
      frame "Scale" {
        n185 = Variant To Data(type=0, Variant=w464) -> (data=w460:i32)  [unwired: 1 in, 1 out]
        n186 = Get Date/Time In Seconds() -> (seconds since 1Jan1904=w466:timestamp)
        n187 = Equal To 0?(x=w460) -> (x = 0?=w461:bool)
        n188 = To Double Precision Float(number=w466) -> (double precision float=w465:dbl)
        n189 = Select(t=2, s=w461, f=0) -> (s? t:f=w459:i32)
        n190 = Subtract(x=w465, y=w460) -> (x-y=w462:dbl)
        n191 = property on="Waveform Chart" class="WFChart (strict)"("XScale.Maximum"=w465, "XScale.Minimum"=w462, "XScale.ScaleFit"=w459) -> ()  [unwired: 2 in, 2 out]
      }
      frame Default {
        # "Case not handled"
        n192 = xnode "Error Ring"("parameter 0"=w472) -> ("error out"=w473:errorcluster)
        n193 = call <vilib>:"Simple Error Handler.vi"("error in (no error)"=w473) -> ()  [unwired: 4 in, 5 out]
      }
    }
    n194 = case shown="1, Default" w203 {
      selector: w203 -> [w213 _]
      tunnel: w199 -> [w215 w321]
      tunnel: w198 -> [w217 w323]
      tunnel: [w216 w323] -> w202
      tunnel: w200 -> [w214 _]
      tunnel: w197 -> [w212 w322]
      tunnel: [w211 w322] -> w196
      tunnel: [w210 w321] -> w193
      frame 1, Default {
        # "Executes after \"Add\", updating the value for the user selected control"
        n195 = case shown="\"CT\"" w212 {
          selector: w212 -> [w226 w240 w254 w271 w303 w313]
          tunnel: [w226 w240 w254 w271 w303 w313] -> w211
          tunnel: w217 -> [w225 w241 w255 w272 w304 w314]
          tunnel: w213 -> [w227 w239 w253 w270 w302 w311]
          tunnel: [w224 w238 w252 w269 w301 w312] -> w216
          tunnel: w214 -> [w230 w244 w258 w262 w297 _]
          tunnel: w215 -> [w229 w243 w257 w265 w298 w306]
          tunnel: [w219 w233 w247 w261 w293 w306] -> w210
          frame "FWD", Default {
            n196 = call "Value adder.vi"("Array"=w225, "Enum"=w226, "value"=w227, "Max Limit"=i16 350) -> ("output array"=w224:i16[], "Limited value"=w218:i16)
            n197 = global write "global variables.vi" "FWD"(w218) -> ()
            n198 = call "PFG600 update value.vi"("Value"=w218, "Command"="\u0000A") -> ("Text"=w223:string, "Hex"=w222:string)
            n199 = property on="Vorwartsleistung (W)" class="Bool (strict)"("BoolText.Text"=w223) -> ()  [unwired: 2 in, 2 out]
            n200 = Bundle("PFG", "Hex"=w222) -> (w220:cluster{string, "Hex":string})  [unwired: 1 in]
            n201 = Enqueue Element(queue=w230, element=w220, error in (no error)=w229) -> (error out=w219:errorcluster)  [unwired: 1 in, 2 out]
          }
          frame "CT" {
            n202 = call "Value adder.vi"("Array"=w241, "Enum"=w240, "value"=w239, "Max Limit"=i16 1000) -> ("output array"=w238:i16[], "Limited value"=w232:i16)
            n203 = global write "global variables.vi" "CT"(w232) -> ()
            n204 = call "PFG600 update value.vi"("Value"=w232, "Command"="\u0001E") -> ("Text"=w237:string, "Hex"=w235:string)
            n205 = property on="CT" class="Bool (strict)"("BoolText.Text"=w237) -> ()  [unwired: 2 in, 2 out]
            n206 = Bundle("PFG", "Hex"=w235) -> (w234:cluster{string, "Hex":string})  [unwired: 1 in]
            n207 = Enqueue Element(queue=w244, element=w234, error in (no error)=w243) -> (error out=w233:errorcluster)  [unwired: 1 in, 2 out]
          }
          frame "CL" {
            n208 = call "Value adder.vi"("Array"=w255, "Enum"=w254, "value"=w253, "Max Limit"=i16 1000) -> ("output array"=w252:i16[], "Limited value"=w246:i16)
            n209 = call "PFG600 update value.vi"("Value"=w246, "Command"="\u0001F") -> ("Text"=w248:string, "Hex"=w250:string)
            n210 = global write "global variables.vi" "CL"(w246) -> ()
            n211 = property on="CL" class="Bool (strict)"("BoolText.Text"=w248) -> ()  [unwired: 2 in, 2 out]
            n212 = Bundle("PFG", "Hex"=w250) -> (w249:cluster{string, "Hex":string})  [unwired: 1 in]
            n213 = Enqueue Element(queue=w258, element=w249, error in (no error)=w257) -> (error out=w247:errorcluster)  [unwired: 1 in, 2 out]
          }
          frame "Ar" {
            # "Sets Ar unless gas boost is active"
            n214 = call "Value adder.vi"("Array"=w272, "Enum"=w271, "value"=w270, "Max Limit"=i16 700) -> ("output array"=w269:i16[], "Limited value"=w267:i16)
            n215 = Divide(x=w267, y=10.0) -> (x/y=w260:dbl)
            n216 = global write "global variables.vi" "Ar"(w260) -> ()
            n217 = Number To Fractional String(number=w260, precision (6)=i16 1) -> (F-format string=w264:string)  [unwired: 2 in]
            n218 = property on="GAS Boost" class="Bool (strict)"() -> ("Value"=w263:bool)  [unwired: 2 in, 2 out]
            n219 = property on="Argon (SCCM)" class="Bool (strict)"("BoolText.Text"=w264) -> ()  [unwired: 2 in, 2 out]
            n220 = case shown="False" w263 {
              tunnel: w264 -> [w281 _]
              tunnel: w262 -> [w280 w284]
              tunnel: [w279 w284] -> _
              tunnel: w265 -> [w274 w283]
              tunnel: [w278 w283] -> w261
              frame False {
                n221 = Concatenate Strings("SP1," ("string"), w281) -> (w277:string)
                n222 = Bundle("PR", w277) -> (w275:cluster{string, string})  [unwired: 1 in]
                n223 = Enqueue Element(queue=w280, element=w275, error in (no error)=w274) -> (queue out=w279:refnum<queue>, error out=w278:errorcluster)  [unwired: 1 in, 1 out]
              }
              frame True {
              }
            }
          }
          frame "O2" {
            # "Sets O2 and opens valve if value is larger than 0"
            n224 = call "Value adder.vi"("Array"=w304, "Enum"=w303, "value"=w302, "Max Limit"=i16 200) -> ("output array"=w301:i16[], "Limited value"=w287:i16)
            n225 = Divide(x=w287, y=10.0) -> (x/y=w285:dbl)
            n226 = Greater Than 0?(x=w287) -> (x > 0?=w286:bool)
            n227 = global write "global variables.vi" "O2"(w285) -> ()
            n228 = Number To Fractional String(number=w285, precision (6)=i16 1) -> (F-format string=w296:string)  [unwired: 2 in]
            n229 = property on="Sauerstioff (SCCM)" class="Bool (strict)"("BoolText.Text"=w296) -> ()  [unwired: 2 in, 2 out]
            n230 = Concatenate Strings("AC2," ("string"), w296, ",ON" ("string")) -> (w290:string)
            n231 = Select(t=w290, s=w286, f="AC2,0,OFF") -> (s? t:f=w288:string)
            n232 = Bundle("PR", w288) -> (w294:cluster{string, string})  [unwired: 1 in]
            n233 = Enqueue Element(queue=w297, element=w294, error in (no error)=w298) -> (error out=w293:errorcluster)  [unwired: 1 in, 2 out]
          }
          frame "Timer" {
            n234 = case shown="0, Default" w311 {
              selector: w311 -> [w318 w320]
              tunnel: [w319 w320] -> w315
              frame 0, Default {
                n235 = Multiply(x=w318, y=6) -> (x*y=w319:i32)
              }
              frame -1, 1 {
              }
            }
            n236 = call "Value adder.vi"("Array"=w314, "Enum"=w313, "value"=w315, "Max Limit"=i16 10800) -> ("output array"=w312:i16[], "Limited value"=w310:i16)
            n237 = Format Date/Time String(time format string (%c)="%H:%M:%S", seconds (now)=w310, UTC format=TRUE) -> (date/time string=w307:string)
            n238 = property on="Timer" class="Bool (strict)"("BoolText.Text"=w307) -> ()  [unwired: 2 in, 2 out]
          }
        }
      }
      frame 0 {
        # "Does nothing  for cases different than \"Add\""
      }
    }
  }
  n239 = while {
    tunnel: w1 -> [w490]
    tunnel: w2 -> [w489]
    stop <- "Stop" stop-if-true
    # "Timer Loop"
    n240 = local read "RS232"() -> (w488:bool)
    n241 = case shown="True" "TimerOn" {
      frame False {
      }
      frame True {
        n242 = local read "Endzeit"() -> (w523:timestamp)
        n243 = Get Date/Time In Seconds() -> (seconds since 1Jan1904=w522:timestamp)
        n244 = Subtract(x=w523, y=w522) -> (x-y=w517:dbl)
        n245 = Round To Nearest(number=w517) -> (nearest integer value=w516:dbl)
        n246 = Format Date/Time String(time format string (%c)="%H:%M:%S", seconds (now)=w517, UTC format=TRUE) -> (date/time string=w518:string)
        n247 = property on="Timer" class="Bool (strict)"("BoolText.Text"=w518) -> ()  [unwired: 2 in, 2 out]
        n248 = Less Or Equal To 0?(x=w516) -> (x <= 0?=w521:bool)
        n249 = case shown="True" w521 {
          frame True {
            w524 = FALSE ("Value (Signaling)")
            n250 = property on="TimerOn" class="Bool (strict)"("Val(Sgnl)"=w524) -> ()  [unwired: 2 in, 2 out]
            n251 = property on="RF Quelle" class="Bool (strict)"("Val(Sgnl)"=w524) -> ()  [unwired: 2 in, 2 out]
          }
          frame False {
          }
        }
      }
    }
    n252 = local read "RF Quelle"() -> (w486:bool)
    n253 = Not(x=w488) -> (.not. x?=w487:bool)
    n254 = And(x=w486, y=w487) -> (x .and. y?=w485:bool)
    n255 = case shown="True" w485 {
      tunnel: w490 -> [_ w503]
      tunnel: w489 -> [_ w498]
      frame False {
      }
      frame True {
        w500 = "PFG"
        n256 = Bundle(w500, "Input"="\u0000Ò\u0000\u0000") -> (w502:cluster{string, "Input":string})  [unwired: 1 in]
        n257 = local read "Matchbox-Modus"() -> (w497:bool)
        n258 = Bundle(w500, "Input"="\u0000Ô\u0000\u0000") -> (w499:cluster{string, "Input":string})  [unwired: 1 in]
        n259 = Enqueue Element(queue=w503, element=w502, error in (no error)=w498) -> (queue out=w506:refnum<queue>, error out=w505:errorcluster)  [unwired: 1 in, 1 out]
        n260 = Enqueue Element(queue=w506, element=w499, error in (no error)=w505) -> (queue out=w495:refnum<queue>, error out=w496:errorcluster)  [unwired: 1 in, 1 out]
        n261 = case shown="True" w497 {
          tunnel: w496 -> [_ w514]
          tunnel: w495 -> [_ w515]
          frame False {
          }
          frame True {
            w509 = "PFG"
            n262 = Bundle(w509, "Input"="\u0001Õ\u0000\u0000") -> (w510:cluster{string, "Input":string})  [unwired: 1 in]
            n263 = Bundle(w509, "Input"="\u0001Ö\u0000\u0000") -> (w507:cluster{string, "Input":string})  [unwired: 1 in]
            n264 = Enqueue Element(queue=w515, element=w510, error in (no error)=w514) -> (queue out=w513:refnum<queue>, error out=w512:errorcluster)  [unwired: 1 in, 1 out]
            n265 = Enqueue Element(queue=w513, element=w507, error in (no error)=w512) -> ()  [unwired: 1 in, 3 out]
          }
        }
      }
    }
    n266 = Get Date/Time In Seconds() -> (seconds since 1Jan1904=→"Time":timestamp)
    n267 = Wait Until Next ms Multiple(millisecond multiple=u32 1000 ("milliseconds to wait")) -> ()  [unwired: 1 out]
  }
  n268 = while {
    tunnel: w2 -> [w529]
    tunnel: w1 -> [w530]
    tunnel: w47 -> [w540]
    tunnel: w46 -> [w539]
    tunnel: [w537] -> w45
    tunnel: [w538] -> w44
    tunnel: w25 -> [w535]
    tunnel: w24 -> [w534]
    tunnel: [w533] -> w23
    tunnel: [w532] -> w22
    tunnel: [w527] -> w11
    tunnel: [w526] -> w12
    stop <- w525 stop-if-true
    # "Instrument  communication loop"
    n269 = Dequeue Element(queue=w530, error in (no error)=w529) -> (queue out=w527:refnum<queue>, element=w528:T2, error out=w526:errorcluster)  [unwired: 1 in, 1 out]
    n270 = Unbundle(w528) -> ("Message"=w536:string, "Message Data"=w531:variant)
    n271 = case shown="\"PFG\"" w536 {
      tunnel: w540 -> [w544 w548 w570 w607]
      tunnel: w539 -> [w543 w547 w569 w608]
      tunnel: [w543 w547 w558 w608] -> w538
      tunnel: [w544 w548 w557 w607] -> w537
      tunnel: w535 -> [w542 w545 w554 w611]
      tunnel: w534 -> [w541 w546 w555 w610]
      tunnel: [w541 w546 w555 w609] -> w533
      tunnel: [w542 w545 w554 w606] -> w532
      tunnel: w531 -> [_ _ w553 w604]
      tunnel: [_ TRUE _ _] -> w525
      frame Default {
      }
      frame "Exit" {
      }
      frame "PFG" {
        n272 = Variant To Data(type="\u0000\u0000\u0000\u0000", Variant=w553) -> (data=w551:string)  [unwired: 1 in, 1 out]
        n273 = call "PFG600 5Byte checksum.vi"("Input"=w551) -> ("Output"=w550:string)
        "PFG600" <- w550
        n274 = VISA Write(VISA resource name=w569, write buffer=w550, error in (no error)=w570) -> (VISA resource name out=w572:refnum<visa-resource-name>, return count=w565:u32, error out=w571:errorcluster)
        n275 = VISA Read(VISA resource name=w572, byte count=w565, error in (no error)=w571) -> (VISA resource name out=w559:refnum<visa-resource-name>, read buffer=w568:string, error out=w556:errorcluster)  [unwired: 1 out]
        "Antwort" <- w568
        n276 = String To Byte Array(string=w568) -> (unsigned byte array=w564:u8[])
        "unsigned byte array" <- w564
        n277 = Index Array(array=w564, index=1) -> (element=w566:u8)
        n278 = Index Array(array=w564, index=0) -> (element=w562:u8)
        n279 = case shown="85" w566 {
          tunnel: w564 -> [_ w579 w585 w592 w598]
          frame Default {
          }
          frame 85 {
            n280 = Index Array(array=w579, index=2) -> (element=w582:u8)
            n281 = Index Array(array=w579, index=3) -> (element=w583:u8)
            n282 = Join Numbers(hi=w582, lo=w583) -> ((hi.lo)=w584:u16)
            n283 = global write "global variables.vi" "CT"(w584) -> ()
          }
          frame 86 {
            n284 = Index Array(array=w585, index=2) -> (element=w588:u8)
            n285 = Index Array(array=w585, index=3) -> (element=w589:u8)
            n286 = Join Numbers(hi=w588, lo=w589) -> ((hi.lo)=w590:u16)
            n287 = global write "global variables.vi" "CL"(w590) -> ()
          }
          frame 82 {
            n288 = Index Array(array=w592, index=2) -> (element=w596:u8)
            n289 = Index Array(array=w592, index=3) -> (element=w594:u8)
            n290 = Join Numbers(hi=w596, lo=w594) -> ((hi.lo)=w591:u16)
            "DC Spannung (V)" <- w591
            n291 = global write "global variables.vi" "DC"(w591) -> ()
          }
          frame 84 {
            n292 = Index Array(array=w598, index=2) -> (element=w602:u8)
            n293 = Index Array(array=w598, index=3) -> (element=w600:u8)
            n294 = Join Numbers(hi=w602, lo=w600) -> ((hi.lo)=w597:u16)
            "REF Leistung (W)" <- w597
            n295 = global write "global variables.vi" "REF"(w597) -> ()
          }
        }
        n296 = Greater?(x=w562, y=u8 1) -> (0:w560:bool)
        n297 = case shown="True" w560 {
          tunnel: w559 -> [w574 w578]
          tunnel: w556 -> [w573 w577]
          tunnel: [w573 w576] -> w557
          tunnel: [w574 w575] -> w558
          frame False {
          }
          frame True {
            # "RS232 Error"
            n298 = VISA Clear(VISA resource name=w578, error in (no error)=w577) -> (VISA resource name out=w575:refnum<visa-resource-name>, error out=w576:errorcluster)
          }
        }
      }
      frame "PR" {
        n299 = Variant To Data(type="", Variant=w604) -> (data=w603:string)  [unwired: 1 in, 1 out]
        "PR4000" <- w603
        n300 = VISA Write(VISA resource name=w611, write buffer=w603, error in (no error)=w610) -> (VISA resource name out=w606:refnum<visa-resource-name>, error out=w609:errorcluster)  [unwired: 1 out]
      }
    }
  }
  n301 = while {
    shift-right: [w621] -> w5
    shift-left: w7 -> [w623]
    shift-right: [w620] -> w4
    shift-left: w6 -> [w622]
    stop <- w618 stop-if-true
    # "Metrics loop"
    n302 = local read "RF Quelle"() -> (w613:bool)
    n303 = local read "Gas"() -> (w614:bool)
    n304 = Or(x=w613, y=w614) -> (x .or. y?=w612:bool)
    n305 = call "Prepare metrics.vi"("LOG Gas"=w614, "LO G RF"=w613) -> ("Metrics"=w619:cluster{string, "O2":dbl}[])
    n306 = call-poly "Send Graphite Metrics (Polymorphic).vi"("error in (no error)"=w622, "Metriics"=w619, "TCP Network Connection in"=w623) -> ("error out"=w620:errorcluster, "TCP Network Connection out"=w621:refnum<k5>)  [unwired: 6 in, 1 out]
    n307 = Select(t=u32 1000 ("milliseconds to wait"), s=w612, f=u32 5000 ("milliseconds to wait")) -> (s? t:f=w615:u32)
    n308 = Wait Until Next ms Multiple(millisecond multiple=w615) -> ()  [unwired: 1 out]
    n309 = local read "Stop"() -> (w618:bool)
  }
  n310 = TCP Close Connection(connection ID=w5, error in (no error)=w4) -> (error out=w3:errorcluster)  [unwired: 1 in, 1 out]
  n311 = call <vilib>:"Simple Error Handler.vi"("error in (no error)"=w3) -> ()  [unwired: 4 in, 5 out]
  n312 = Release Queue(queue=w14, error in (no error)=w13) -> ()  [unwired: 1 in, 3 out]
  n313 = Release Queue(queue=w11, error in (no error)=w12) -> ()  [unwired: 1 in, 3 out]
  n314 = VISA Close(VISA resource name=w44, error in (no error)=w45) -> (error out=w43:errorcluster)
  n315 = VISA Close(VISA resource name=w22, error in (no error)=w23) -> (error out=w42:errorcluster)
  n316 = call <vilib>:"Simple Error Handler.vi"("error in (no error)"=w43) -> ()  [unwired: 4 in, 5 out]
  n317 = call <vilib>:"Simple Error Handler.vi"("error in (no error)"=w42) -> ()  [unwired: 4 in, 5 out]
  n318 = Merge Errors(w30, w18) -> (w29:errorcluster)
  n319 = call <vilib>:"Simple Error Handler.vi"("error in (no error)"=w29) -> ()  [unwired: 4 in, 5 out]
